vi "test.vi"() -> ()   [LabVIEW 2013]
uses:
  lv_lib/CHR34XXX.lvlib
panel:
  in  "通道号":u8 max=23 step=1
  out "devId":i32
  in  "Mode":u8
  in  "pstRsdcb":T1
  out "Exit":bool
  in  "退出":bool
  in  "(10us)":u32=100000
  in  "定时发送":bool
  out "RxFlag":bool
  in  "开始接收":bool
  out "RxData(Hex)":string
  in  "发送":bool
  out "布尔":bool
  in  "TxData(Hex)":string
  in  "通道号":u8 max=23 step=1
  # "Mode：通道模式，0 表示 232 模式，1 表示 422 模式，2 表示 485 模式 \nBaudRate：波特率\nRS232：75~500Kbps\nRS422/485：75~2.4Mbps\nByteSize：数据位长度，取值范围为 5~8\nStopBits：停止位个数，取值范围为 0~2\n取值为 0 时，表示 1 位停止位(ByteSize 取值为 5~8)\n取值为 1 时，表示 1.5 位停止位(ByteSize 取值为 5)\n取值为 2 时，表示 2 位停止位(ByteSize 取值为 6~8)\nParity：校验方式，取值范围为 0~4\n0：无校验，1：奇校验，2：偶校验，3：Mark 校验，4：Space 校验"
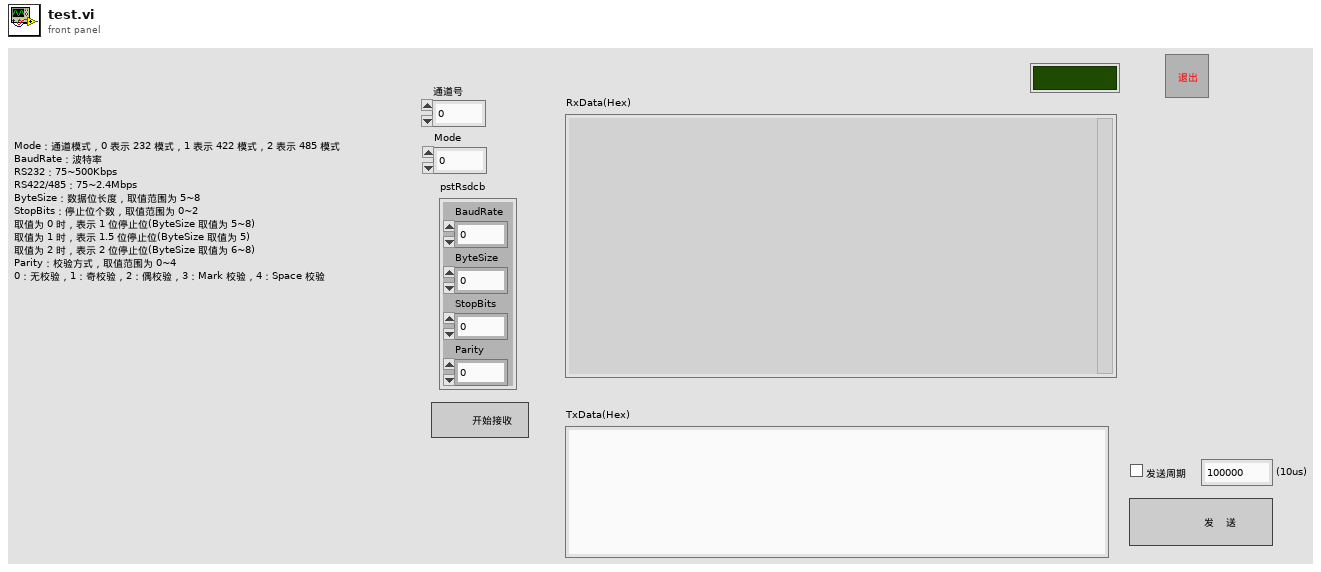
[diagram p1: front panel]
types:
  T1 = cluster{"BaudRate":u32, "ByteSize":u32, "StopBits":u32, "Parity":u32}
  T2 = enum8{"Enabled", "Disabled", "Disabled and Grayed Out"}
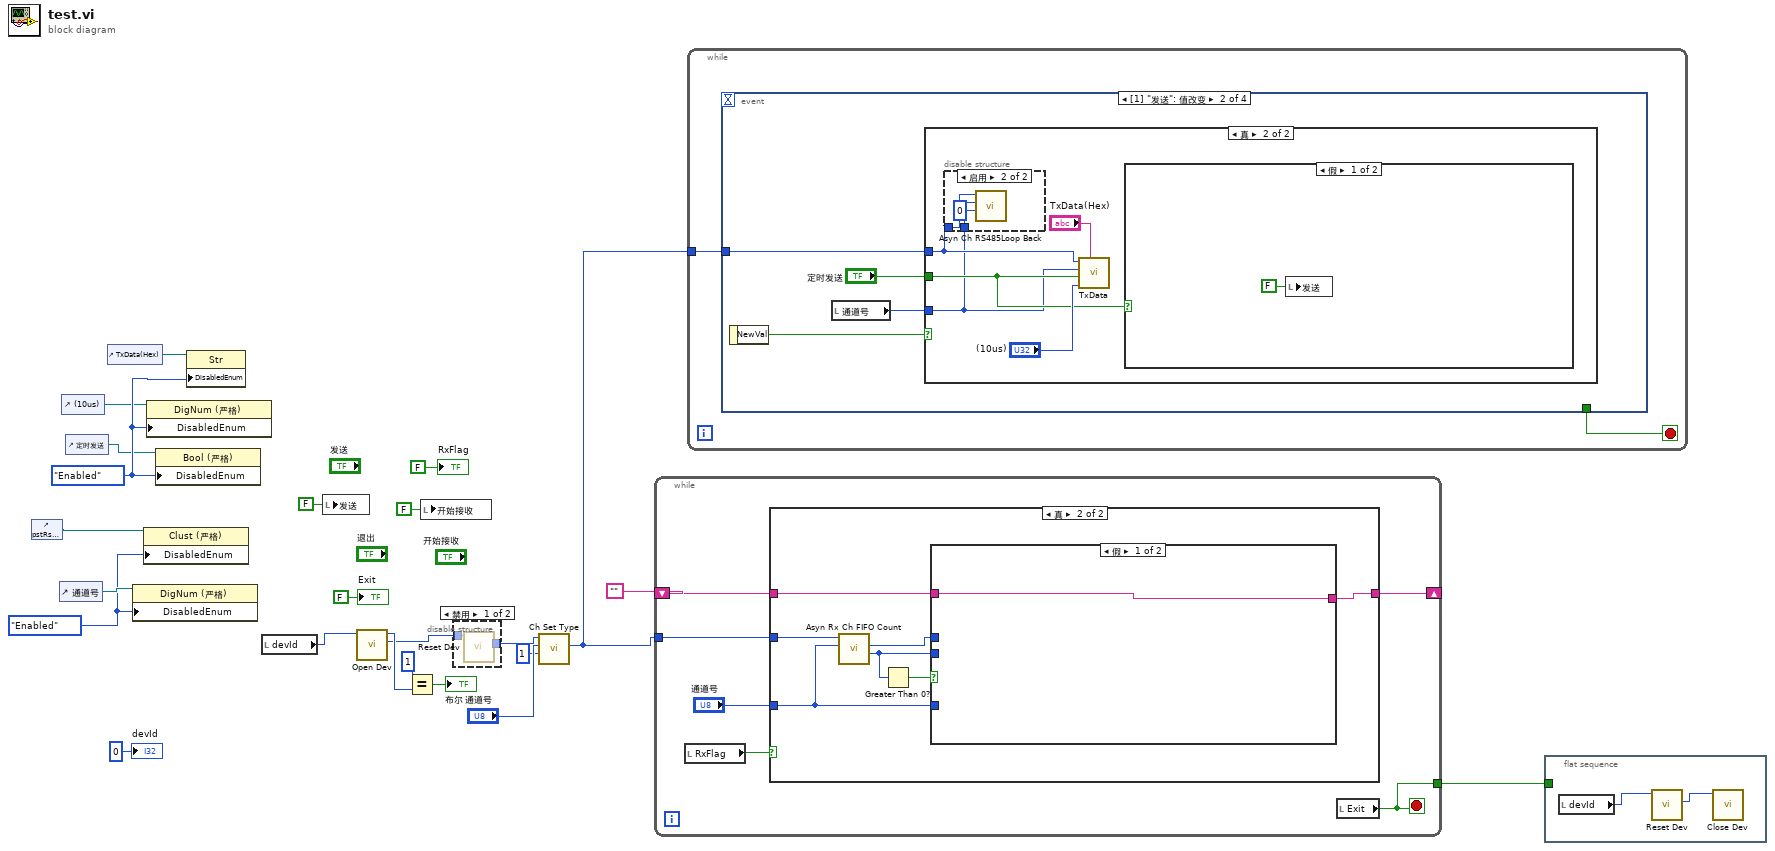
[diagram p0: block diagram]
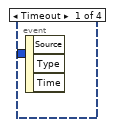
[diagram p3: hidden frame]
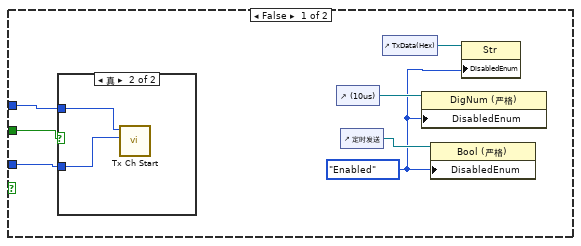
[diagram p4: hidden frame]
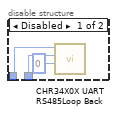
[diagram p6: hidden frame]
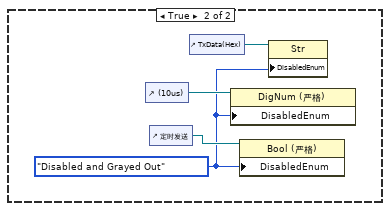
[diagram p7: hidden frame]
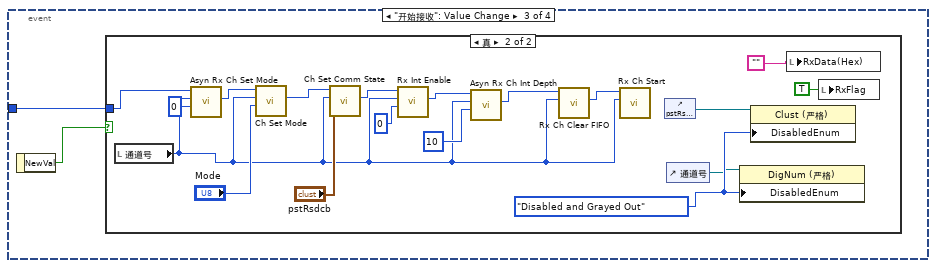
[diagram p8: hidden frame]
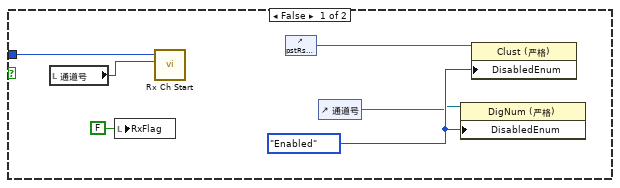
[diagram p9: hidden frame]
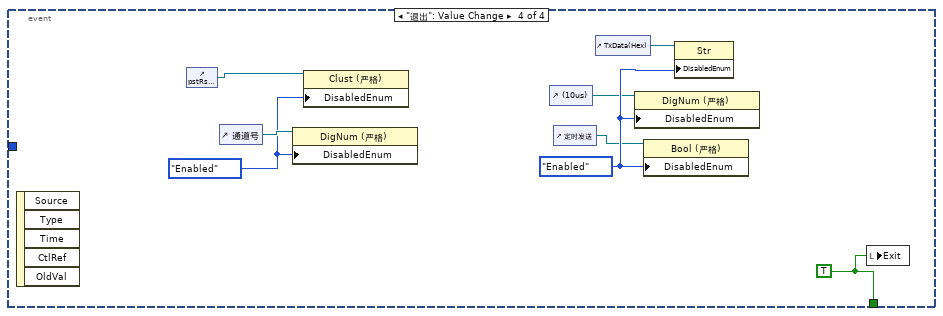
[diagram p10: hidden frame]
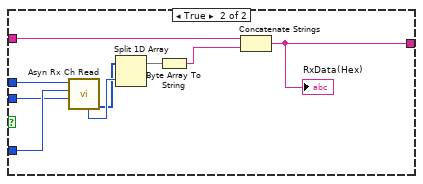
[diagram p12: hidden frame]
diagram:
  w13 = T2."Enabled" ("禁用")
  w14 = T2."Enabled" ("禁用")
  n1 = control-ref of="pstRsdcb"() -> (w8:refnum<vi>)
  n2 = control-ref of="通道号"() -> (w15:refnum<vi>)
  n3 = control-ref of="(10us)"() -> (w10:refnum<vi>)
  n4 = control-ref of="定时发送"() -> (w11:refnum<vi>)
  n5 = control-ref of="TxData(Hex)"() -> (w12:refnum<vi>)
  n6 = property class="DigNum (严格)"(reference=w15, "DisabledEnum"=w14) -> ()  [unwired: 1 in, 2 out]
  n7 = property class="Clust (严格)"(reference=w8, "DisabledEnum"=w14) -> ()  [unwired: 1 in, 2 out]
  n8 = property class="DigNum (严格)"(reference=w10, "DisabledEnum"=w13) -> ()  [unwired: 1 in, 2 out]
  n9 = property class="Bool (严格)"(reference=w11, "DisabledEnum"=w13) -> ()  [unwired: 1 in, 2 out]
  n10 = property class="Str"(reference=w12, "DisabledEnum"=w13) -> ()  [unwired: 1 in, 2 out]
  n11 = local read "devId"() -> (w7:i32)
  n12 = local write "发送"(FALSE ("发送")) -> ()
  n13 = call "Open Dev.vi"("devId in"=w7) -> ("devId out"=w9:i32, "function return"=w18:i32)  [unwired: 9 in]
  n14 = Equal?(x=1, y=w18) -> (x = y?=→"布尔":bool)
  n15 = local write "开始接收"(FALSE ("开始接收")) -> ()
  n16 = disable-structure shown="禁用" {
    disable-tunnel: w9 -> [w25 _]
    disable-tunnel: [w24 _] -> w4
    frame Disabled {
      n17 = call "Reset Dev.vi"("devId"=w25) -> ("devId out"=w24:i32)  [unwired: 9 in, 1 out]
    }
    frame Enabled {
    }
  }
  n18 = call "Ch Set Type.vi"("Type"=u8 1, "Channel"="通道号", "devId"=w4) -> ("devId out"=w1:i32)  [unwired: 7 in, 1 out]
  n19 = while {
    tunnel: w1 -> [w31]
    shift-right: [w30] -> _
    shift-left: "" -> [w29]
    tunnel: [w26] -> w16
    stop <- w26 stop-if-true
    n20 = local read "RxFlag"() -> (w27:bool)
    n21 = case shown="真" w27 {
      tunnel: w31 -> [_ w39]
      tunnel: "通道号" -> [_ w37]
      tunnel: [w32 w35] -> w30
      tunnel: w29 -> [w32 w34]
      frame False {
      }
      frame True {
        n22 = call "Asyn Rx Ch FIFO Count.vi"("Channel"=w37, "devId"=w39) -> ("pCount out"=w36:u32, "devId out"=w33:i32)  [unwired: 7 in, 1 out]
        n23 = Greater Than 0?(x=w36) -> (x > 0?=w38:bool)
        n24 = case shown="假" w38 {
          tunnel: w33 -> [_ w49]
          tunnel: w37 -> [_ w48]
          tunnel: w36 -> [_ w47]
          tunnel: [w40 w42] -> w35
          tunnel: w34 -> [w40 w44]
          frame False {
          }
          frame True {
            n25 = call "Asyn Rx Ch Read.vi"("Length"=w47, "Channel"=w48, "devId"=w49) -> ("pBuffer out"=w41:u8[], "pReturned out"=w46:u32)  [unwired: 5 in, 2 out]
            n26 = Split 1D Array(array=w41, index=w46) -> (first subarray=w45:u8[])  [unwired: 1 out]
            n27 = Byte Array To String(unsigned byte array=w45) -> (string=w43:string)
            n28 = Concatenate Strings(w44, w43) -> (w42:string)
            "RxData(Hex)" <- w42
          }
        }
      }
    }
    n29 = local read "Exit"() -> (w26:bool)
  }
  n30 = while {
    tunnel: w1 -> [w51]
    stop <- w50 stop-if-true
    n31 = event shown="[1] \"发送\": 值改变" {
      selector: _ -> [_ _ _ _]
      dyn-events: _ -> [_ _ _ _]
      timeout: _ -> [_ _ _ _]
      tunnel: w51 -> [_ w55 w82 _]
      tunnel: [_ _ _ w114] -> w50
      event Timeout {
        n32 = event-data() -> ()  [unwired: 1 in, 3 out]
      }
      event "发送": Value Change {
        n33 = event-data() -> ("NewVal"=w54:bool)  [unwired: 1 in]
        n34 = local read "通道号"() -> (w53:u8)
        n35 = case shown="真" w54 {
          tunnel: w55 -> [w62 w66]
          tunnel: w53 -> [w61 w65]
          tunnel: "定时发送" -> [w60 w67]
          frame False {
            w56 = T2."Enabled" ("禁用")
            n36 = case shown="真" w60 {
              tunnel: w62 -> [_ w64]
              tunnel: w61 -> [_ w63]
              frame False {
              }
              frame True {
                n37 = call "Tx Ch Start.vi"("Channel"=w63, "devId"=w64) -> ()  [unwired: 8 in, 2 out]
              }
            }
            n38 = control-ref of="(10us)"() -> (w59:refnum<vi>)
            n39 = control-ref of="定时发送"() -> (w58:refnum<vi>)
            n40 = control-ref of="TxData(Hex)"() -> (w57:refnum<vi>)
            n41 = property class="DigNum (严格)"(reference=w59, "DisabledEnum"=w56) -> ()  [unwired: 1 in, 2 out]
            n42 = property class="Bool (严格)"(reference=w58, "DisabledEnum"=w56) -> ()  [unwired: 1 in, 2 out]
            n43 = property class="Str"(reference=w57, "DisabledEnum"=w56) -> ()  [unwired: 1 in, 2 out]
          }
          frame True {
            n44 = disable-structure shown="启用" {
              disable-tunnel: w66 -> [w72 w75]
              disable-tunnel: w65 -> [w71 w74]
              frame Disabled {
                n45 = call "CHR34X0X UART RS485Loop Back.vi"("Enabled"=0 ("bl485SelChk"), "Channel"=w71, "devId"=w72) -> ()  [unwired: 7 in, 2 out]
              }
              frame Enabled {
                n46 = call "Asyn Ch RS485Loop Back.vi"("Enabled"=0, "Channel"=w74, "devId"=w75) -> ()  [unwired: 7 in, 2 out]
              }
            }
            n47 = call "TxData.vi"("TxData(Hex)"="TxData(Hex)", "Period(10us)"="(10us)", "定时发送"=w67, "通道号"=w65, "Handle"=w66) -> ()  [unwired: 7 in]
            n48 = case shown="假" w67 {
              frame False {
                n49 = local write "发送"(FALSE ("发送")) -> ()
              }
              frame True {
                w77 = T2."Disabled and Grayed Out" ("禁用")
                n50 = control-ref of="(10us)"() -> (w80:refnum<vi>)
                n51 = control-ref of="定时发送"() -> (w79:refnum<vi>)
                n52 = control-ref of="TxData(Hex)"() -> (w78:refnum<vi>)
                n53 = property class="DigNum (严格)"(reference=w80, "DisabledEnum"=w77) -> ()  [unwired: 1 in, 2 out]
                n54 = property class="Bool (严格)"(reference=w79, "DisabledEnum"=w77) -> ()  [unwired: 1 in, 2 out]
                n55 = property class="Str"(reference=w78, "DisabledEnum"=w77) -> ()  [unwired: 1 in, 2 out]
              }
            }
          }
        }
      }
      event "开始接收": Value Change {
        n56 = event-data() -> ("NewVal"=w81:bool)  [unwired: 1 in]
        n57 = case shown="真" w81 {
          tunnel: w82 -> [w88 w92]
          frame False {
            w85 = T2."Enabled" ("禁用")
            n58 = local read "通道号"() -> (w87:u8)
            n59 = local write "RxFlag"(FALSE ("RxFlag")) -> ()
            n60 = call "Rx Ch Start.vi"("Channel"=w87, "devId"=w88) -> ()  [unwired: 8 in, 2 out]
            n61 = control-ref of="pstRsdcb"() -> (w83:refnum<vi>)
            n62 = control-ref of="通道号"() -> (w84:refnum<vi>)
            n63 = property class="DigNum (严格)"(reference=w84, "DisabledEnum"=w85) -> ()  [unwired: 1 in, 2 out]
            n64 = property class="Clust (严格)"(reference=w83, "DisabledEnum"=w85) -> ()  [unwired: 1 in, 2 out]
          }
          frame True {
            w103 = T2."Disabled and Grayed Out" ("禁用")
            n65 = local read "通道号"() -> (w89:u8)
            n66 = call "Asyn Rx Ch Set Mode.vi"("Mode"=u8 0, "Channel"=w89, "devId"=w92) -> ("devId out"=w90:i32)  [unwired: 7 in, 1 out]
            n67 = call "Ch Set Mode.vi"("Mode"="Mode", "Channel"=w89, "devId"=w90) -> ("devId out"=w100:i32)  [unwired: 7 in, 1 out]
            n68 = call "Ch Set Comm State.vi"("pstRsdcb"="pstRsdcb", "Channel"=w89, "devId"=w100) -> ("devId out"=w98:i32)  [unwired: 6 in, 2 out]
            n69 = call "Rx Int Enable.vi"("Enabled"=0, "Channel"=w89, "devId"=w98) -> ("devId out"=w95:i32)  [unwired: 7 in, 1 out]
            n70 = call "Asyn Rx Ch Int Depth.vi"("Depth"=10 ("Enabled"), "Channel"=w89, "devId"=w95) -> ("devId out"=w94:i32)  [unwired: 7 in, 1 out]
            n71 = call "Rx Ch Clear FIFO.vi"("Channel"=w89, "devId"=w94) -> ("devId out"=w101:i32)  [unwired: 8 in, 1 out]
            n72 = call "Rx Ch Start.vi"("Channel"=w89, "devId"=w101) -> ()  [unwired: 8 in, 2 out]
            n73 = control-ref of="pstRsdcb"() -> (w96:refnum<vi>)
            n74 = control-ref of="通道号"() -> (w102:refnum<vi>)
            n75 = property class="DigNum (严格)"(reference=w102, "DisabledEnum"=w103) -> ()  [unwired: 1 in, 2 out]
            n76 = property class="Clust (严格)"(reference=w96, "DisabledEnum"=w103) -> ()  [unwired: 1 in, 2 out]
            n77 = local write "RxData(Hex)"("") -> ()
            n78 = local write "RxFlag"(TRUE ("RxFlag")) -> ()
          }
        }
      }
      event "退出": Value Change {
        w111 = T2."Enabled" ("禁用")
        w112 = T2."Enabled" ("禁用")
        w114 = TRUE
        n79 = event-data() -> ()  [unwired: 1 in, 5 out]
        n80 = control-ref of="pstRsdcb"() -> (w107:refnum<vi>)
        n81 = control-ref of="通道号"() -> (w113:refnum<vi>)
        n82 = property class="DigNum (严格)"(reference=w113, "DisabledEnum"=w112) -> ()  [unwired: 1 in, 2 out]
        n83 = property class="Clust (严格)"(reference=w107, "DisabledEnum"=w112) -> ()  [unwired: 1 in, 2 out]
        n84 = control-ref of="(10us)"() -> (w108:refnum<vi>)
        n85 = control-ref of="定时发送"() -> (w109:refnum<vi>)
        n86 = control-ref of="TxData(Hex)"() -> (w110:refnum<vi>)
        n87 = property class="DigNum (严格)"(reference=w108, "DisabledEnum"=w111) -> ()  [unwired: 1 in, 2 out]
        n88 = property class="Bool (严格)"(reference=w109, "DisabledEnum"=w111) -> ()  [unwired: 1 in, 2 out]
        n89 = property class="Str"(reference=w110, "DisabledEnum"=w111) -> ()  [unwired: 1 in, 2 out]
        n90 = local write "Exit"(w114) -> ()
      }
    }
  }
  n91 = flat-sequence {
    tunnel: w16 -> [_]
    frame #0 {
      n92 = local read "devId"() -> (w115:i32)
      n93 = call "Reset Dev.vi"("devId"=w115) -> ("devId out"=w116:i32)  [unwired: 9 in, 1 out]
      n94 = call "Close Dev.vi"("devId"=w116) -> ()  [unwired: 9 in, 2 out]
    }
  }
  "RxFlag" <- FALSE ("RxFlag")
  "Exit" <- FALSE ("Exit")
  "devId" <- 0 ("devId")
